vi "Initialize.vi"(5 "components directory":path, 7 "options":T1={"FIFO Options"={"Infinite Timeouts"=FALSE}, "Thread Options"={"Show FP On Call"=FALSE, "Close FP After Call"=FALSE, "Allow Debugging"=FALSE}, "Plugin Options"={"Default Components"=FALSE}, "Performance Options"={"Measure Period"=FALSE, "Measure Rx/Tx Duration"=FALSE}, "Data Server Options"={"Enable Data Server"=FALSE, "Period"=50}} {"Data Server Options"."Period" format="%d ms"}, 8 "error in (no error)":errorcluster, 10 "Framework Configuration":refnum<class "Framework Configuration.lvclass">=refnum, 11 "VeriStand DSF in":refnum<class "VeriStand DSF.lvclass">=refnum) -> (0 "error out":errorcluster, 3 "VeriStand DSF out":refnum<class "VeriStand DSF.lvclass">)   [LabVIEW 2021, in "DSF Engine.lvlib" / "VeriStand DSF.lvclass"]
uses:
  VeriStand DSF.lvclass
  Includes/DSF Core.lvlibp/Classes/Framework/Framework Options.ctl
  Includes/DSF Core.lvlibp/Typedefs/DSF Performance Options.ctl
  Includes/DSF Core.lvlibp/Typedefs/DSF FIFO Options.ctl
  Includes/DSF Core.lvlibp/Classes/Thread/Thread Options.ctl
  Includes/DSF Core.lvlibp/Typedefs/DSF Plugin Options.ctl
  Includes/DSF Core.lvlibp/Classes/Framework/Data Server Options.ctl
  Includes/DSF Core.lvlibp/Classes/Configuration/Core/Framework/Framework Configuration.lvclass
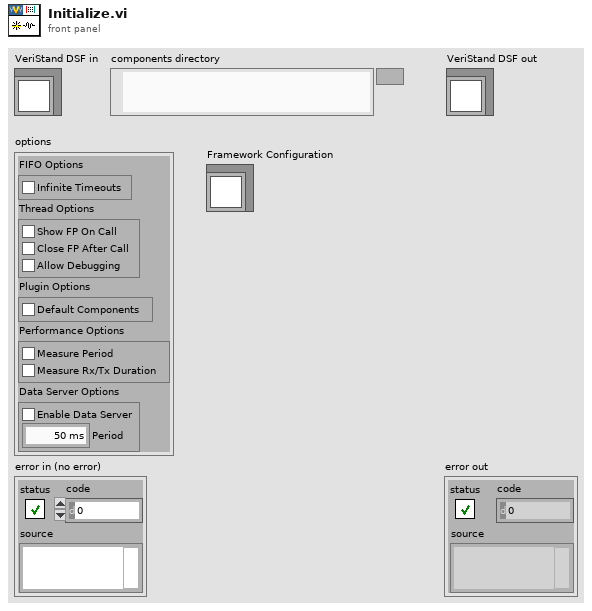
[diagram p1: front panel]
types:
  T1 = typedef "DSF Core.lvlibp/Framework.lvclass/Framework Options.ctl" = cluster{"FIFO Options":T2, "Thread Options":T3, "Plugin Options":T4, "Performance Options":T5, "Data Server Options":T6}
  T2 = typedef "DSF Core.lvlibp/Framework.lvclass/DSF FIFO Options.ctl" = cluster{"Infinite Timeouts":bool}
  T3 = typedef "DSF Core.lvlibp/Thread.lvclass/Thread Options.ctl" = cluster{"Show FP On Call":bool, "Close FP After Call":bool, "Allow Debugging":bool}
  T4 = typedef "DSF Core.lvlibp/Framework.lvclass/DSF Plugin Options.ctl" = cluster{"Default Components":bool}
  T5 = typedef "DSF Core.lvlibp/DSF Performance Options.ctl" = cluster{"Measure Period":bool, "Measure Rx/Tx Duration":bool}
  T6 = typedef "DSF Core.lvlibp/Framework.lvclass/Data Server Options.ctl" = cluster{"Enable Data Server":bool, "Period":u32}
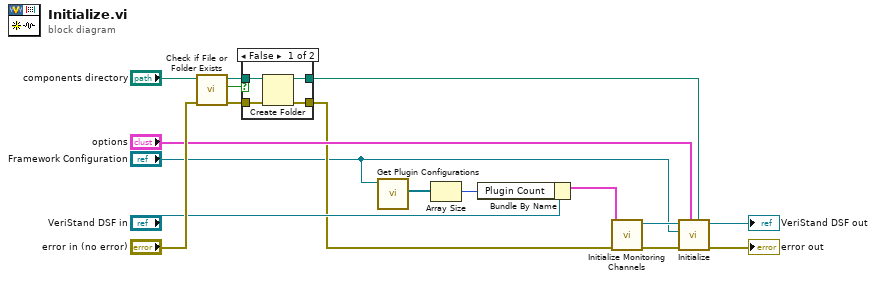
[diagram p0: block diagram]
diagram:
  n1 = call <vilib>:"Check if File or Folder Exists.vi"("error in (no error)"="error in (no error)", "path"="components directory") -> ("error out"=w11:errorcluster, "file or folder exists?"=w9:bool, "dup path"=w10:path)  [unwired: 7 in]
  n2 = case shown="False" w9 {
    tunnel: w11 -> [w21 w22]
    tunnel: [w20 w22] -> w4
    tunnel: w10 -> [w19 w23]
    tunnel: [w18 w23] -> w7
    frame False {
      n3 = Create Folder(path (use dialog)=w19, error in=w21) -> (created path=w18:path, error out=w20:errorcluster)  [unwired: 1 in, 1 out]
    }
    frame True {
    }
  }
  n4 = call "Get Plugin Configurations.vi"("Framework Configuration in"="Framework Configuration") -> ("Plugin Configurations"=w6:refnum<class "Plugin Configuration.lvclass">[])  [unwired: 8 in, 2 out]
  n5 = Array Size(array=w6) -> (size(s)=w13:i32)
  n6 = Bundle By Name(cluster="VeriStand DSF in", "Plugin Count"=w13) -> (w5:cluster{})
  n7 = call "Initialize Monitoring Channels.vi"("error in (no error)"=w4, "VeriStand Data Sharing Framework in"=w5) -> ("error out"=w2:errorcluster, "VeriStand Data Sharing Framework out"=w3:refnum<class "VeriStand DSF.lvclass">)  [unwired: 8 in]
  n8 = call-parent "Initialize.vi"("components directory (default)"=w7, "framework options"="options", "error in (no error)"=w2, "Framework Configuration"="Framework Configuration", "Framework in"=w3) -> ("error out"=→"error out":errorcluster, "Framework out"=→"VeriStand DSF out":refnum<class "VeriStand DSF.lvclass">)  [unwired: 5 in]
